vi "APP Close Interface.vi"(0 "APP Setup":T1, 11 "Error In (no error)":errorcluster) -> (15 "Error Out":errorcluster)   [LabVIEW 2011]
uses:
  Type Defs/APP Application Setup Cluster.ctl
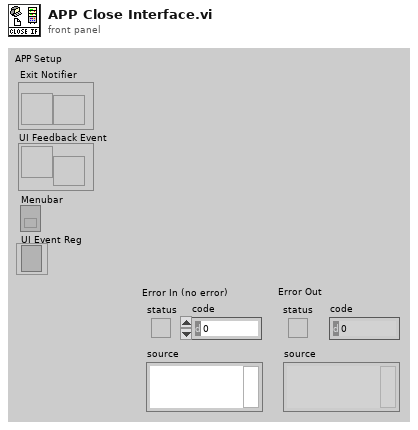
[diagram p1: front panel]
types:
  T1 = typedef "APP Application Setup Cluster.ctl" = cluster{"Menubar":refnum<k9>, "Exit Notifier":refnum<notifier>, "UI Feedback Event":refnum<user-event>, "UI Event Reg":refnum<event-registration>}
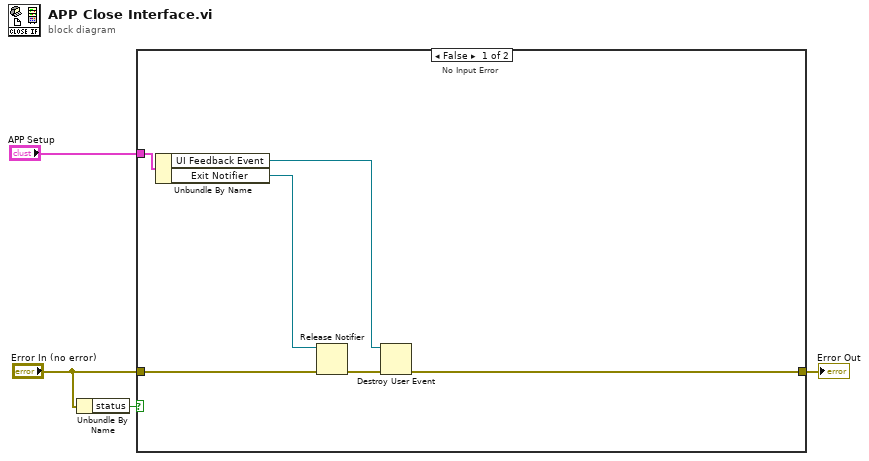
[diagram p0: block diagram]
diagram:
  n1 = Unbundle By Name("Error In (no error)") -> ("status"=w4:bool)
  n2 = case shown="False" w4 {
    tunnel: [w5 w11] -> w3
    tunnel: "Error In (no error)" -> [w9 w11]
    tunnel: "APP Setup" -> [w10 _]
    frame False {
      # "No Input Error"
      n3 = Unbundle By Name(w10) -> ("UI Feedback Event"=w7:refnum<user-event>, "Exit Notifier"=w6:refnum<notifier>)
      n4 = Release Notifier(notifier=w6, error in (no error)=w9) -> (error out=w8:errorcluster)  [unwired: 1 in, 2 out]
      n5 = Destroy User Event(user event=w7, error in=w8) -> (error out=w5:errorcluster)
    }
    frame True {
      # "Input Error"
    }
  }
  "Error Out" <- w3
